vi "006 Panel Init.vi"(8 "error in (no error)":errorcluster caption="Error In") -> (0 "error out":errorcluster caption="Error Out")   [LabVIEW 2020]
uses:
  006 System Gloabl.vi
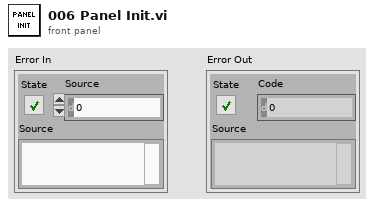
[diagram p1: front panel]
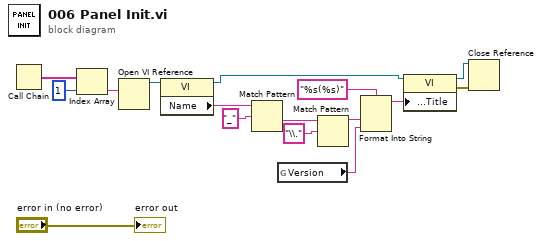
[diagram p0: block diagram]
diagram:
  n1 = Call Chain() -> (call chain=w16:string[])
  n2 = Index Array(array=w16, index=1 ("索引")) -> (element=w15:string)
  n3 = Open VI Reference(vi path=w15) -> (vi reference=w13:refnum<vi>)  [unwired: 5 in, 1 out]
  n4 = property class="VI"(reference=w13) -> (reference out=w4:refnum<vi>, "Name"=w12:string)  [unwired: 1 in, 1 out]
  n5 = Match Pattern(string=w12, regular expression="_" ("正则表达式")) -> (after substring=w10:string)  [unwired: 1 in, 3 out]
  n6 = global read "006 System Gloabl.vi" "Version"() -> (w6:string)
  n7 = Match Pattern(string=w10, regular expression="\\." ("正则表达式")) -> (before substring=w7:string)  [unwired: 1 in, 3 out]
  n8 = Format Into String(format string="%s(%s)" ("格式字符串"), w7, w6) -> (resulting string=w3:string)  [unwired: 2 in, 1 out]
  n9 = property class="VI"(reference=w4, "Front Panel.Title"=w3) -> (reference out=w1:refnum<vi>, error out=w2:errorcluster)  [unwired: 1 in]
  n10 = Close Reference(reference=w1, error in (no error)=w2) -> ()  [unwired: 1 out]
  "error out" <- "error in (no error)"
